vi "enumerateStaticDependencies.vi"(8 "error in (no error)":errorcluster, 11 "Instrument":refnum<class "Instrument.lvclass">) -> (0 "error out":errorcluster, 2 "Static Dependencies":refnum<class "Dependency.lvclass">[](array[class]), 3 "Instrument out":refnum<class "Instrument.lvclass">)   [LabVIEW 2016, in "Instrument.lvclass"]
doc: "JKI State Machine Objects (SMO) 1.3.0.56\nJKI - JKI\nCopyright (c) 2017, JKI"
uses:
  Instrument.lvclass
  <vilib>/JKI/JKI SMO/Dependency/Dependency.lvclass
  levylab_util_remote/src/SMOs/RemoteControl.STM/RemoteControl.STM.lvclass
  C:/Program Files (x86)/National Instruments/LabVIEW 2016/vi.lib/JKI/JKI SMO/SMO/SMO.lvclass
  Logger/Logger.lvclass
  levylab_util_remote/src/SMOs/RemoteControl/RemoteControl.lvclass
  <vilib>/JKI/JKI SMO/SMO/SMO.lvclass
panel:
  # "For instructions on how to use the JKI State Machine Objects, examples and video tutorials, visit:\nhttp://jki.net/state-machine-objects/\n\nJKI State Machine Objects™\nhttp://jki.net/state-machine-objects/\nCopyright (C) 2005-2015, JKI <info@jki.net>\nALL RIGHTS RESERVED"
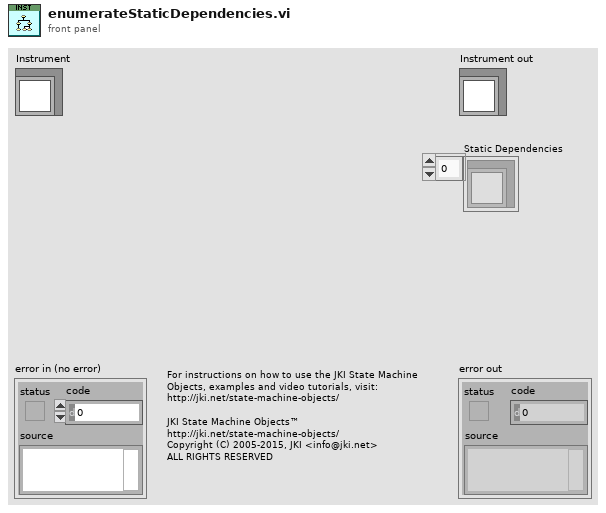
[diagram p1: front panel]
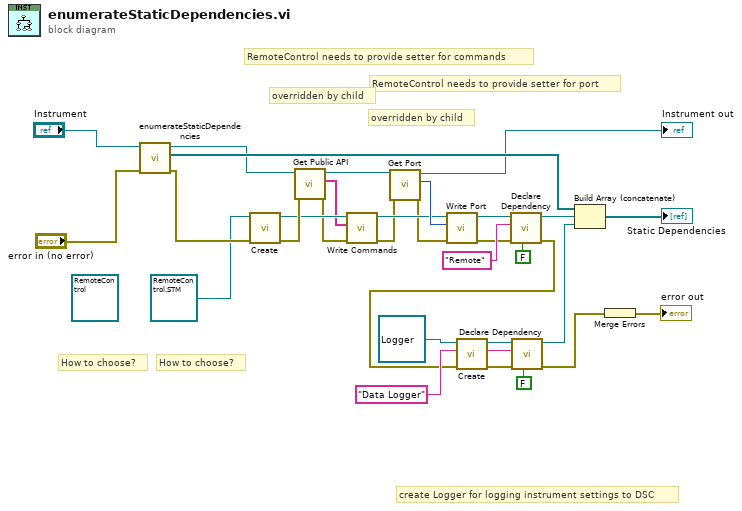
[diagram p0: block diagram]
diagram:
  (unwired) refnum<class "RemoteControl.lvclass"> refnum ("RemoteControl.lvclass")
  # "create Logger for logging instrument settings to DSC"
  # "How to choose?"
  # "How to choose?"
  # "RemoteControl needs to provide setter for port"
  # "RemoteControl needs to provide setter for commands"
  # "overridden by child"
  # "overridden by child"
  n1 = call-parent "enumerateStaticDependencies.vi"("error in (no error)"="error in (no error)", "SMO"="Instrument") -> ("error out"=w24:errorcluster, "Static Dependencies"=w28:refnum<class "Dependency.lvclass">[], "SMO out"=w4:refnum<class "Instrument.lvclass">)  [unwired: 7 in]
  n2 = call <vilib>:"Create.vi"("error in (no error)"=w24, "SMO"=refnum<class "RemoteControl.STM.lvclass"> refnum ("RemoteControl.STM.lvclass")) -> ("error out"=w23:errorcluster, "SMO out"=w21:refnum<class "RemoteControl.STM.lvclass">)  [unwired: 7 in, 1 out]
  n3 = call-dynamic "Get Public API.vi"("error in (no error)"=w23, "Instrument in"=w4) -> ("error out"=w20:errorcluster, "Commands"=w19:string[], "Instrument out"=w25:refnum<class "Instrument.lvclass">)  [unwired: 7 in]
  n4 = call-dynamic "Write Commands.vi"("error in (no error)"=w20, "Commands"=w19, "RemoteControl in"=w21) -> ("error out"=w15:errorcluster, "RemoteControl out"=w17:refnum<class "RemoteControl.STM.lvclass">)  [unwired: 7 in]
  n5 = call-dynamic "Get Port.vi"("error in (no error)"=w15, "Instrument in"=w25) -> ("error out"=w16:errorcluster, "port"=w18:u32, "Instrument out"=→"Instrument out":refnum<class "Instrument.lvclass">)  [unwired: 7 in]
  n6 = call-dynamic "Write Port.vi"("error in (no error)"=w16, "Port"=w18, "RemoteControl in"=w17) -> ("error out"=w13:errorcluster, "RemoteControl out"=w14:refnum<class "RemoteControl.STM.lvclass">)  [unwired: 7 in]
  n7 = call <vilib>:"Declare Dependency.vi"("Shared Resource (F)"=FALSE, "error in (no error)"=w13, "Name"="Remote", "Type"=w14) -> ("error out"=w1:errorcluster, "Dependency out"=w29:refnum<class "Dependency.lvclass">)  [unwired: 6 in]
  n8 = call <vilib>:"Create.vi"("error in (no error)"=w1, "Subsystem Name (optional)"="Data Logger" ("Name"), "SMO"=refnum<class "Logger.lvclass"> refnum ("Logger.lvclass")) -> ("error out"=w8:errorcluster, "SMO name"=w2:string, "SMO out"=w9:refnum<class "Logger.lvclass">)  [unwired: 6 in]
  n9 = call <vilib>:"Declare Dependency.vi"("Shared Resource (F)"=FALSE, "error in (no error)"=w8, "Name"=w2, "Type"=w9) -> ("error out"=w7:errorcluster, "Dependency out"=w10:refnum<class "Dependency.lvclass">)  [unwired: 6 in]
  n10 = Build Array (concatenate)(w28, w29, w10) -> (→"Static Dependencies":refnum<class "Dependency.lvclass">[])
  n11 = Merge Errors(w7) -> (→"error out":errorcluster)
